vi "LEP_RV_IncBuild_Read.vi"(1 "Rebuild?":bool) -> (0 "Incremental Build?":bool)   [LabVIEW 2011]
uses:
  <vilib>/Platform/EmbProject/Plugins/utilities/LEP_Utilities_GetSetProjectData_Variant.vi
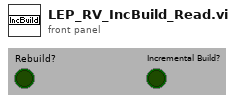
[diagram p1: front panel]
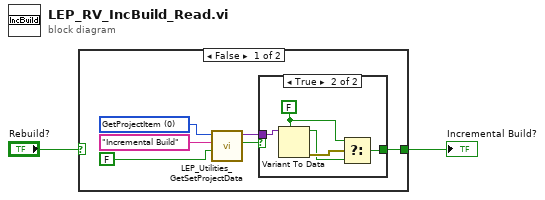
[diagram p0: block diagram]
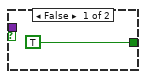
[diagram p2: hidden frame]
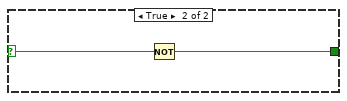
[diagram p3: hidden frame]
diagram:
  n1 = case shown="False" "Rebuild?" {
    selector: "Rebuild?" -> [_ w16]
    tunnel: [w3 w15] -> w1
    frame False {
      w8 = u16 0 items=["GetProjectItem", "SetProjectItem"] ("Command")
      n2 = call-poly <vilib>:"LEP_Utilities_GetSetProjectData.vi"("Variant In"=FALSE, "ItemName"="Incremental Build", "Command"=w8) -> ("Found/Replaced?"=w5:bool, "Variant Out"=w4:variant)  [unwired: 2 in, 5 out]
      n3 = case shown="True" w5 {
        tunnel: w4 -> [_ w14]
        tunnel: [TRUE w10] -> w3
        frame False {
        }
        frame True {
          w12 = FALSE
          n4 = Variant To Data(type=w12, Variant=w14) -> (data=w11:bool, error out=w13:errorcluster)  [unwired: 1 in]
          n5 = Select(t=w12, s=w13, f=w11) -> (s? t:f=w10:bool)
        }
      }
    }
    frame True {
      n6 = Not(x=w16) -> (.not. x?=w15:bool)
    }
  }
  "Incremental Build?" <- w1
